vi "Create-Destroy.vi"(8 "Error In":errorcluster) -> (0 "Error Out":errorcluster)   [LabVIEW 2017, in "Tests.lvlib" / "Session.lvlib"]
uses:
  Session.lvlib
  <vilib>/addons/_JKI Toolkits/Caraya/classes/Test/Test.lvclass
  src/Toolkit/Toolkit.lvlib
  src/Toolkit/API/Session/Session.lvclass
  <vilib>/addons/_JKI Toolkits/Caraya/classes/Assert/Assert.lvclass
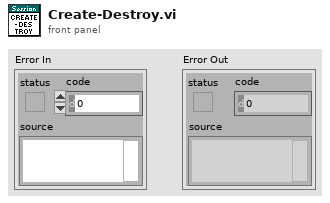
[diagram p1: front panel]
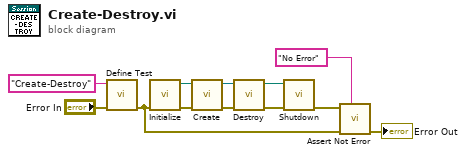
[diagram p0: block diagram]
diagram:
  n1 = call <vilib>:"Define Test.vi"("error in (no error)"="Error In", "Label (VI Title)"="Create-Destroy") -> ("error out"=w2:errorcluster)  [unwired: 9 in]
  n2 = call "Initialize.vi"("Error In"=w2) -> ("Error Out"=w10:errorcluster, "labssh2 Shared Library Out"=w9:path)  [unwired: 9 in]
  n3 = call "Create.vi"("Error In"=w10, "labssh2 Shared Library"=w9) -> ("Error Out"=w7:errorcluster, "Sesssion"=w8:refnum<class "Session.lvclass">)  [unwired: 8 in]
  n4 = call "Destroy.vi"("Error In"=w7, "Session"=w8) -> ("Error Out"=w5:errorcluster, "labssh2 Shared Library"=w6:path)  [unwired: 8 in]
  n5 = call "Shutdown.vi"("Error In"=w5, "labssh2 Shared Library"=w6) -> ("Error Out"=w4:errorcluster)  [unwired: 9 in]
  n6 = call <vilib>:"Assert Not Error.vi"("Label"="No Error", "error in (no error)"=w2, "Not Error?"=w4) -> ("error out"=→"Error Out":errorcluster)  [unwired: 8 in]
